vi "CDF Mechanism Manual.vi"(7 "Description":string, 8 "Command Info In":T1, 11 "Setpoint":dbl) -> (0 "Command Info Out":T1)   [LabVIEW 2015]
uses:
  <vilib>/Rock Robotics/WPI/Framework/Command Status Info.ctl
  <vilib>/Rock Robotics/WPI/Framework/Completion Status.ctl
  <vilib>/Rock Robotics/WPI/Framework/Completion Notifier.ctl
  Implementation/CDF Mechanism Setpoints.ctl
  Implementation/CDF Mechanism Operations.ctl
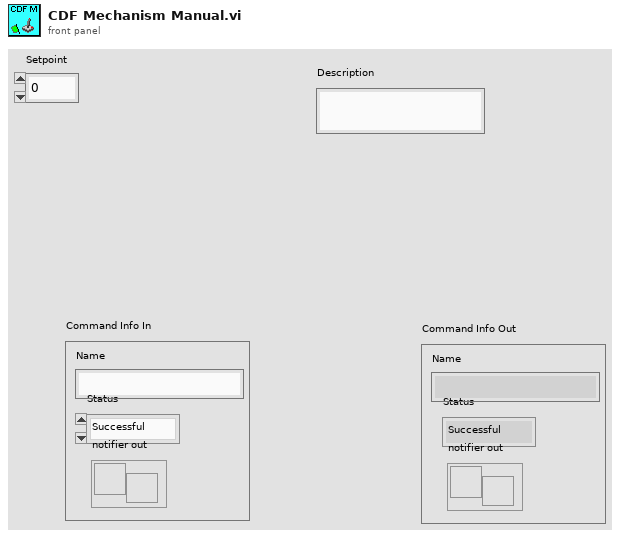
[diagram p1: front panel]
types:
  T1 = typedef "Command Status Info.ctl" = cluster{"Name":string, "Status":T2, "notifier out":T3}
  T2 = typedef "Completion Status.ctl" = enum16{"Successful", "Aborted", "Incomplete"}
  T3 = typedef "Completion Notifier.ctl" = refnum<notifier>
  T4 = typedef "CDF Mechanism Setpoints.ctl" = cluster{"Operation":T5, "Setpoint":dbl, "Duration":dbl, "Setpoint (Top is = True )":bool}
  T5 = typedef "CDF Mechanism Operations.ctl" = enum16{"Reserve", "Read Current", "Immediate", "Idle", "Flip", "Set", "Manual"}
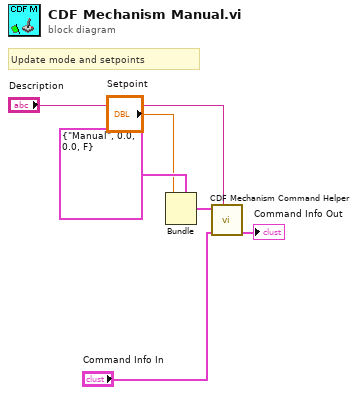
[diagram p0: block diagram]
diagram:
  # "Update mode and setpoints"
  n1 = Bundle(cluster=T4 {"Operation"=enum."Manual", "Setpoint"=0.0, "Duration"=0.0, "Setpoint (Top is = True )"=FALSE} ("SubSystem Data"), "Setpoint"="Setpoint") -> (w2:T4)  [unwired: 3 in]
  n2 = call "CDF Mechanism Command Helper.vi"("Description"="Description", "Command Info In"="Command Info In", "SubSystem Data"=w2) -> ("Command Info Out"=→"Command Info Out":T1)  [unwired: 7 in, 1 out]
